vi "DecoderMessageFlag.vi"(8 "error in":errorcluster, 9 "Array":u8[](array[numeric]) format="%02x") -> (0 "error IO":errorcluster, 2 "array w/ subset deleted":u8[](array[numeric]), 3 "flags":cluster{"id":dbl, "flag":bool})   [LabVIEW 2017]
uses:
  SSL-SOS/Varint Decoder uint32.vi
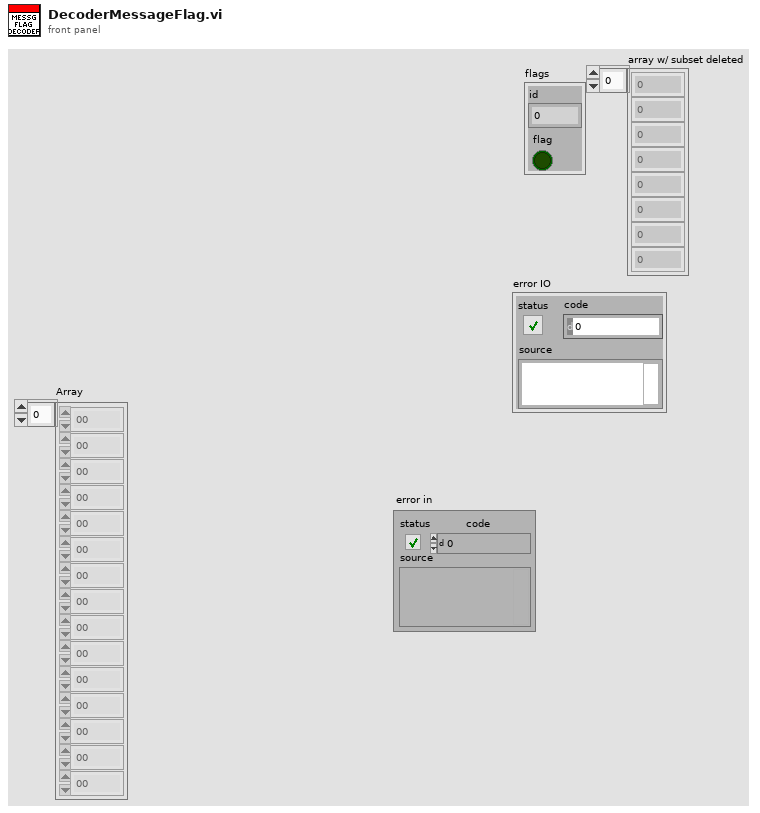
[diagram p1: front panel]
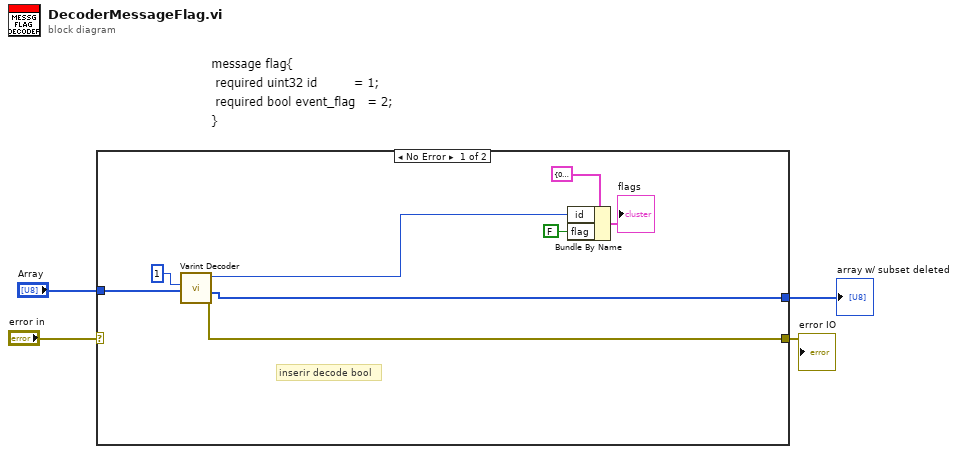
[diagram p0: block diagram]
diagram:
  n1 = case shown="No Error" "error in" {
    selector: "error in" -> [_ w13]
    tunnel: "Array" -> [w12 w14]
    tunnel: [w6 w14] -> w2
    tunnel: [w5 w13] -> w1
    frame No Error {
      # "inserir decode bool"
      n2 = call-poly "Varint Decoder.vi"("Array"=w12, "Key"=1) -> ("error out"=w5:errorcluster, "array w/ subset deleted"=w6:u8[], "Varint"=w8:u32)  [unwired: 6 in, 1 out]
      n3 = Bundle By Name(cluster=cluster{"id":dbl, "flag":bool} {"id"=0.0, "flag"=FALSE} ("flags 2"), "id"=w8, "flag"=FALSE) -> (→"flags":cluster{"id":dbl, "flag":bool})
    }
    frame Error {
    }
  }
  "array w/ subset deleted" <- w2
  "error IO" <- w1
